vi "specify execution settings.vi"(8 "error in":errorcluster, 10 "channels":refnum<class "TBM channel.lvclass">[](array[class]), 11 "fixed channel runtime in":refnum<class "fixed channel runtime.lvclass">) -> (0 "error out":errorcluster, 2 "execution settings":T1, 3 "fixed channel runtime out":refnum<class "fixed channel runtime.lvclass">)   [LabVIEW 2013, in "fixed channel runtime.lvclass"]
uses:
  fixed channel runtime.lvclass
  <vilib>/NI/Tag Bus Module Framework/runtime/execution settings.ctl
  <vilib>/NI/Tag Bus Module Framework/channel/TBM channel.lvclass
  <vilib>/NI/Tag Bus Module Framework/runtime/TBM module execution interface.lvclass
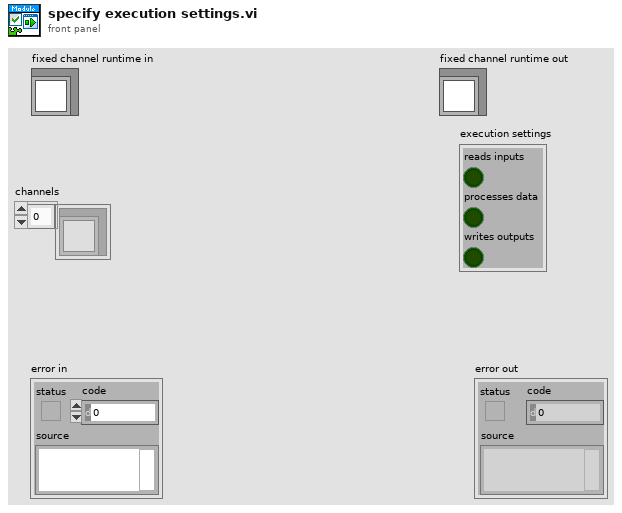
[diagram p1: front panel]
types:
  T1 = typedef "TBM module execution interface.lvclass/execution settings.ctl" = cluster{"reads inputs":bool, "processes data":bool, "writes outputs":bool}
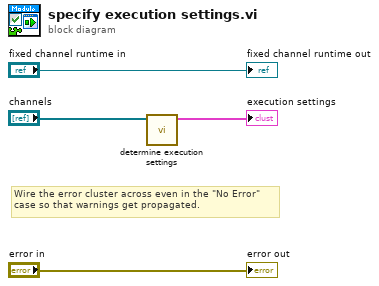
[diagram p0: block diagram]
diagram:
  # "Wire the error cluster across even in the \"No Error\"\ncase so that warnings get propagated."
  n1 = call <vilib>:"determine execution settings.vi"("channels"="channels") -> ("execution settings"=→"execution settings":T1)  [unwired: 10 in]
  "error out" <- "error in"
  "fixed channel runtime out" <- "fixed channel runtime in"
